vi "Rinocloud_get_metadata.vi"(3 "id":string) -> (0 "body":string, 1 "headers":string)   [LabVIEW 2013]
uses:
  Rinocloud_global_variable.vi
  <vilib>/httpClient/POSTBuffer.vi
  <vilib>/httpClient/LabVIEWHTTPClient.lvlib
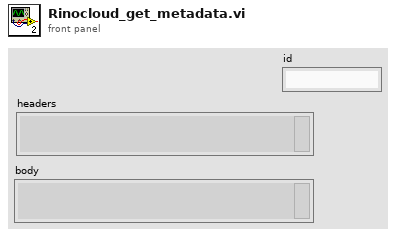
[diagram p1: front panel]
types:
  T1 = typedef "LabVIEWHTTPClient.lvlib/ClientHandle.ctl" = refnum<k1>
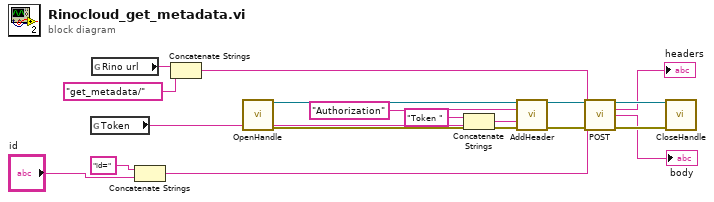
[diagram p0: block diagram]
diagram:
  n1 = global read "Rinocloud_global_variable.vi" "Token"() -> (w10:string)
  n2 = global read "Rinocloud_global_variable.vi" "Rino url"() -> (w16:string)
  n3 = Concatenate Strings("id=" ("value"), "id") -> (w3:string)
  n4 = Concatenate Strings(w16, "get_metadata/" ("Combo Box 2")) -> (w18:string)
  n5 = call <vilib>:"OpenHandle.vi"() -> ("client handle out"=w14:T1, "error out"=w11:errorcluster)  [unwired: 14 in]
  n6 = Concatenate Strings("Token " ("value"), w10) -> (w12:string)
  n7 = call <vilib>:"AddHeader.vi"("client handle"=w14, "header"="Authorization" ("url"), "value"=w12, "error in (no error)"=w11) -> ("client handle out"=w7:T1, "error out"=w6:errorcluster)  [unwired: 10 in]
  n8 = call-poly <vilib>:"POST.vi"("client handle"=w7, "url"=w18, "buffer"=w3, "error in (no error)"=w6) -> ("client handle out"=w9:T1, "headers"=→"headers":string, "body"=→"body":string, "error out"=w8:errorcluster)  [unwired: 8 in]
  n9 = call <vilib>:"CloseHandle.vi"("client handle"=w9, "error in (no error)"=w8) -> ()  [unwired: 13 in, 1 out]
